vi "Do.vi"(8 "error in":errorcluster, 10 "Actor in":refnum<class "Actor.lvclass">, 11 "Update Filter Cycle Params MSG":refnum<class "Update Filter Cycle Params MSG.lvclass">) -> (0 "error out":errorcluster, 2 "Actor out":refnum<class "Actor.lvclass">)   [LabVIEW 2014, in "Controller.lvlib" / "Update Filter Cycle Params MSG.lvclass"]
doc: "(<B>Filename</B>: Actor Framework.lvlib:Message.lvclass:Do.vi)\n\nDefines what a message does when it is received by an actor. Generally, a message instructs an actor to invoke one of its methods. By default, this method does nothing. A child class must override it to define behavior. Create a child class by using the Actor Framework Message Maker dialog box."
uses:
  Update Filter Cycle Params MSG.lvclass
  <vilib>/ActorFramework/Actor/Actor.lvclass
  Update Filter Cycle Params MSG.lvclass/Update Filter Cycle Params MSG.ctl
  Controller.lvclass
  Controller.lvclass/Controller.ctl
  SuperActor/Ex Nested.lvclass/Ex Nested.ctl
  reusable/Switch/Switch.lvclass/Switch.ctl
  reusable/Switch/Write Cycle_.vi
  Accessors/Read Switch DVR.vi
  SuperActor/Read Log Session.vi
  SuperActor/Read CVT Session.vi
  reusable/Switch/Write maxElapseTime.vi
  <userlib>/_Session Fwk/Session - Root.lvclass
  reusable/Switch/Switch.lvclass
  reusable/Session APIs/Session Log/System Log.lvclass
  reusable/Session APIs/CVT/CVT.lvclass
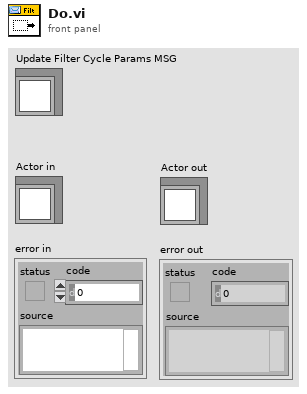
[diagram p1: front panel]
types:
  T1 = typedef "Session - Root.lvclass/Session Handle.ctl" = refnum<data-value>
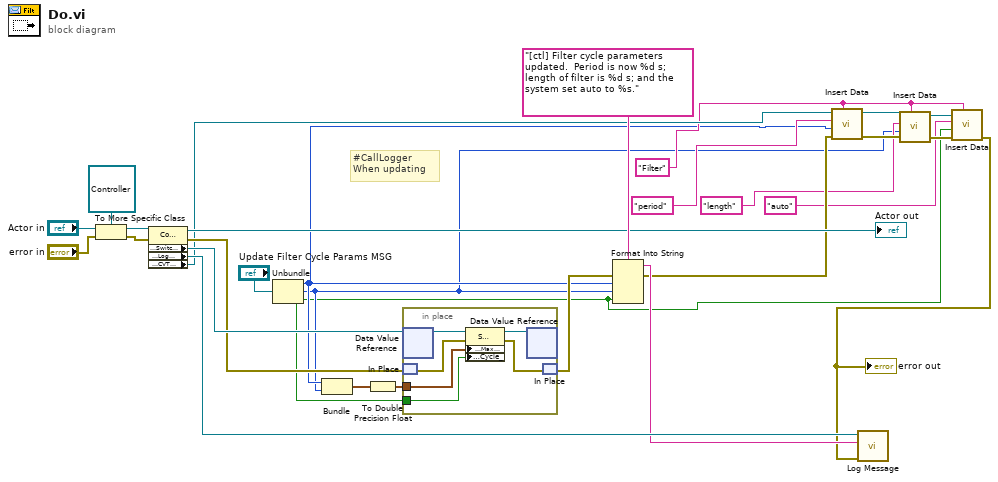
[diagram p0: block diagram]
diagram:
  w11 = "Filter" ("Group")
  # "#CallLogger\nWhen updating"
  n1 = To More Specific Class(target class=refnum<class "Controller.lvclass"> refnum ("Controller.lvlib:Controller"), reference="Actor in", error in="error in") -> (specific class reference=w26:refnum<class "Controller.lvclass">, error out=w25:errorcluster)
  n2 = property class="Controller"(reference=w26, error in=w25) -> (reference out=→"Actor out":refnum<class "Controller.lvclass">, error out=w20:errorcluster, "Accessors:Switch DVR"=w24:refnum<data-value>, "Accessors:Log Session"=w19:T1, "Accessors:CVT Session"=w14:T1)
  n3 = Unbundle("Update Filter Cycle Params MSG") -> (w9:u16, w5:u16, w2:bool)
  n4 = Bundle("Period"=w9, "Length"=w5) -> (w22:cluster{"Period":u16, "Length":u16})  [unwired: 1 in]
  n5 = To Double Precision Float(number=w22) -> (double precision float=w21:cluster{"Period":dbl, "Length":dbl})
  n6 = in-place {
    in-place-border: w21 -> [w33]
    in-place-border: w2 -> [w32]
    n7 = in-place-dvr #1(w24) -> (w35:refnum<class "Switch.lvclass">)  [unwired: 1 out]
    n8 = in-place-match #2(w20) -> (w31:errorcluster)
    n9 = property class="Switch"(reference=w35, error in=w31, "Data Access:Max Elapsed Time"=w33, "Accessors:Cycle_"=w32) -> (reference out=w34:refnum<class "Switch.lvclass">, error out=w30:errorcluster)
    n10 = in-place-dvr #1(w34) -> ()  [unwired: 2 out]
    n11 = in-place-match #2(w30) -> (w15:errorcluster)
  }
  n12 = Format Into String(format string="[ctl] Filter cycle parameters updated.  Period is now %d s; length of filter is %d s; and the system set auto to %s.", error in=w15, w9, w5, w2) -> (resulting string=w17:string, error out=w8:errorcluster)  [unwired: 1 in]
  n13 = call "Insert Data.vi"("tag"=w11, "error in"=w8, "Data"=w9, "Group"="period" ("tag"), "CVT Session In"=w14) -> ("error out"=w7:errorcluster, "CVT Session Out"=w13:T1)  [unwired: 5 in]
  n14 = call "Insert Data.vi"("tag"=w11, "error in"=w7, "Data"=w5, "Group"="length" ("tag"), "CVT Session In"=w13) -> ("error out"=w4:errorcluster, "CVT Session Out"=w12:T1)  [unwired: 5 in]
  n15 = call "Insert Data.vi"("tag"=w11, "error in"=w4, "Data"=w2, "Group"="auto" ("tag"), "CVT Session In"=w12) -> ("error out"=w1:errorcluster)  [unwired: 5 in, 1 out]
  "error out" <- w1
  n16 = call "Log Message.vi"("error in"=w1, "MSG In"=w17, "session in"=w19) -> ()  [unwired: 7 in, 2 out]
